vi "Superlight Control.vi"() -> ()   [LabVIEW 2014]
uses:
  statecontrol.ctl
  <vilib>/LabVIEW Interface for Arduino/Type Defs/Board Type.ctl
  <vilib>/LabVIEW Interface for Arduino/Type Defs/Connection Type.ctl
  <vilib>/LabVIEW Interface for Arduino/Type Defs/Pin Mode.ctl
  <vilib>/LabVIEW Interface for Arduino/Type Defs/Arduino Resource.ctl
  <vilib>/LabVIEW Interface for Arduino/LabVIEW Interface for Arduino.lvlib
panel:
  in  "stop 3":bool
  out "high":bool
  out "low":bool
  in  "Power State":bool
  out "Superlight State":T1
  out "cooldown status":bool
  out "Cooldown Time Left":u32 format="%<%M:%S>t"
  out "superlight status":bool
  out "Cooldown Start Time":u32
  in  "stop 2":bool
  out "Superlight On Start Time":u32
  out "Is the button pressed?":bool
  out "Tab Control":enum32{" On", "Off", "CoolDown"}(tab)
  in  "Off":bool
  # "Low"
  # "High"
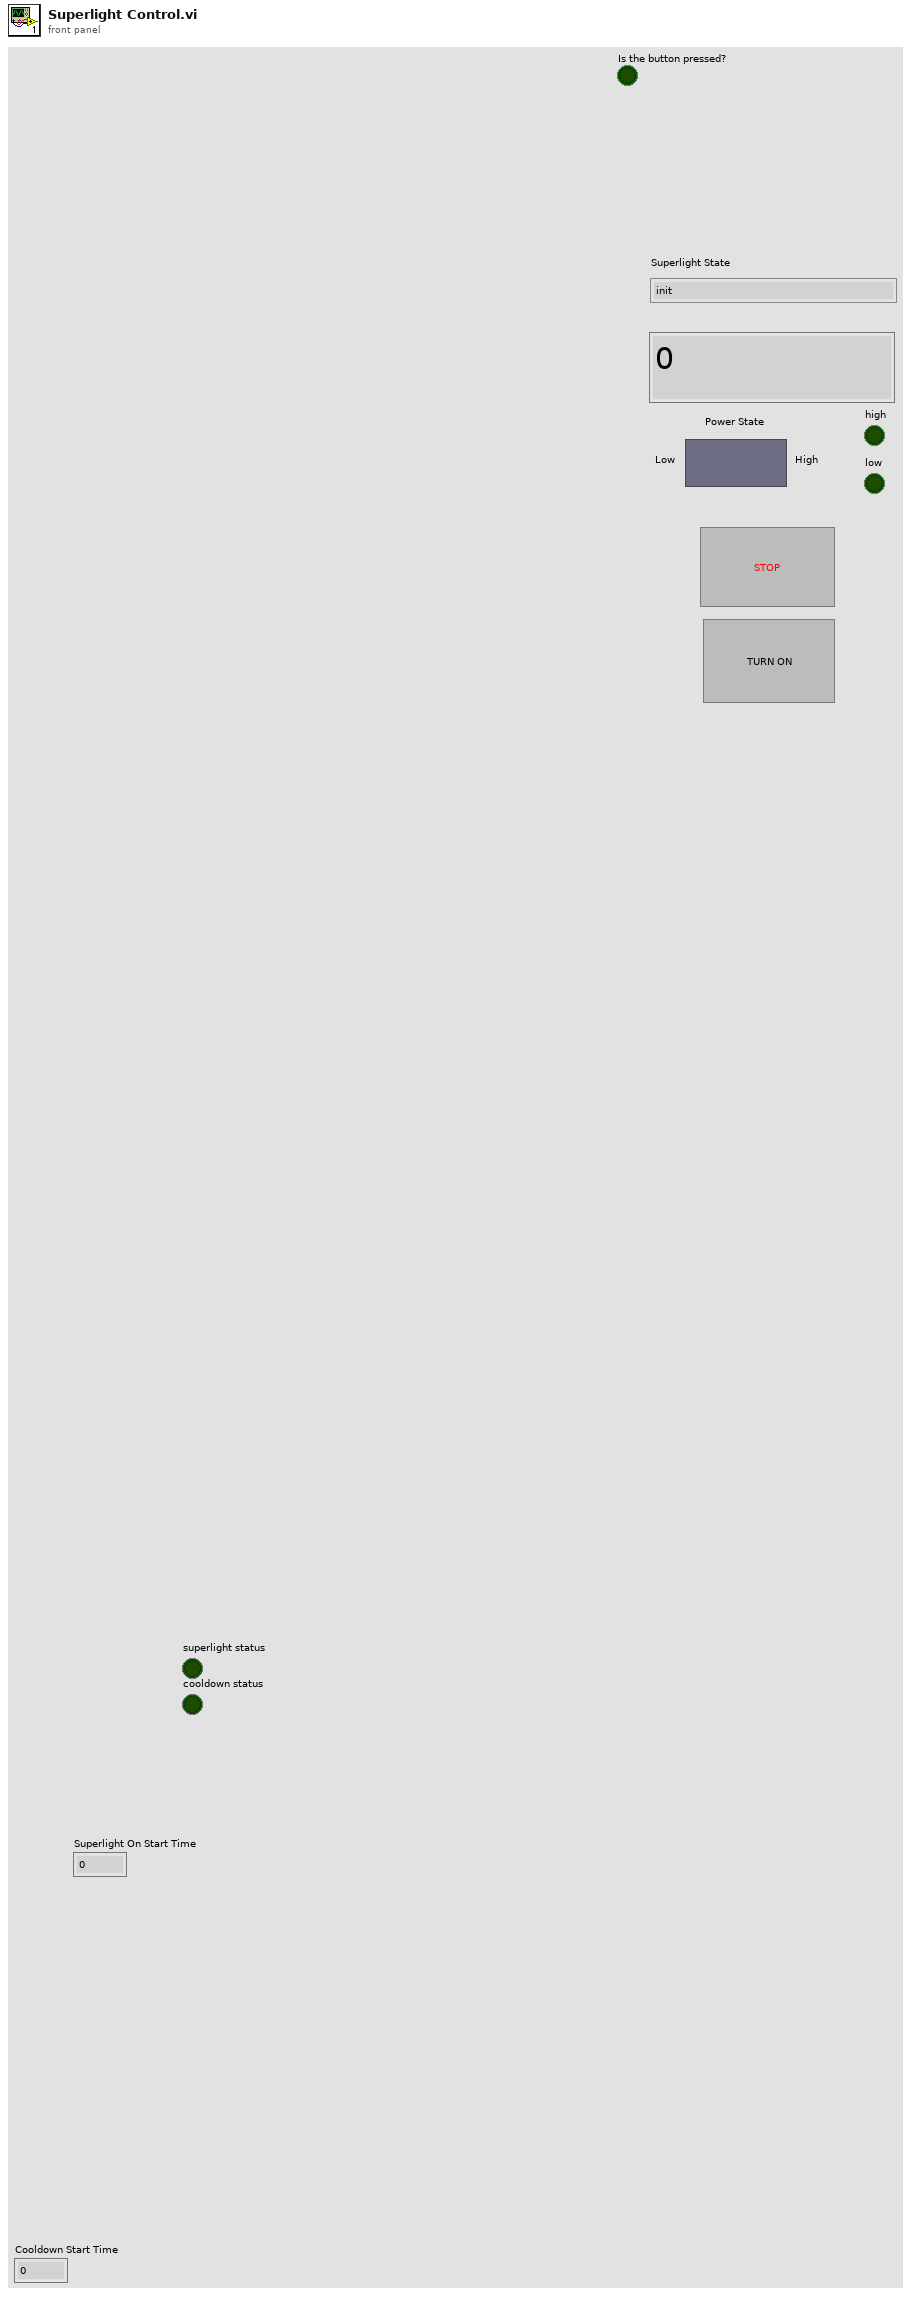
[diagram p1: front panel]
types:
  T1 = typedef "statecontrol.ctl" = enum16{"init", "waiting for trigger", "superlight on", "cooldown", "closing", "shutdown"}
  T2 = typedef "LabVIEW Interface for Arduino.lvlib/Pin Mode.ctl" = enum8{"Input", "Output"}
  T3 = typedef "LabVIEW Interface for Arduino.lvlib/Connection Type.ctl" = enum8{"USB / Serial", "XBEE", "BlueSmirf (Bluetooth)"}
  T4 = typedef "LabVIEW Interface for Arduino.lvlib/Board Type.ctl" = enum16{"Uno", "Dimuelanove w/Atmega 328", "Mega 2560"}
  T5 = typedef "LabVIEW Interface for Arduino.lvlib/Arduino Resource.ctl" = cluster{"VISA resource":refnum<visa-resource-name>, "Board Type":T4, "Connection Type":enum8{"USB / Serial"}, "Bytes Per Packet (15)":u8}
  T6 = enum8{"Enabled", "Disabled", "Disabled and Grayed Out"}
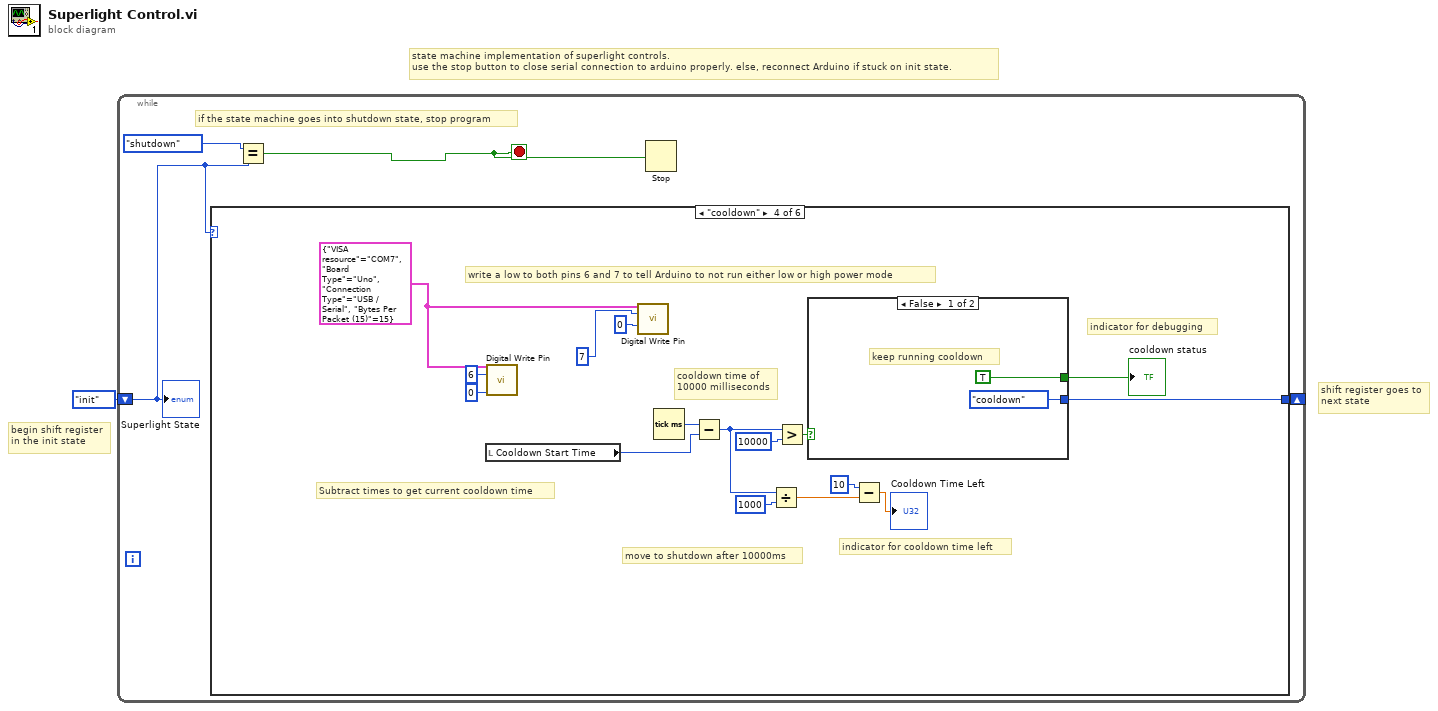
[diagram p0: block diagram]
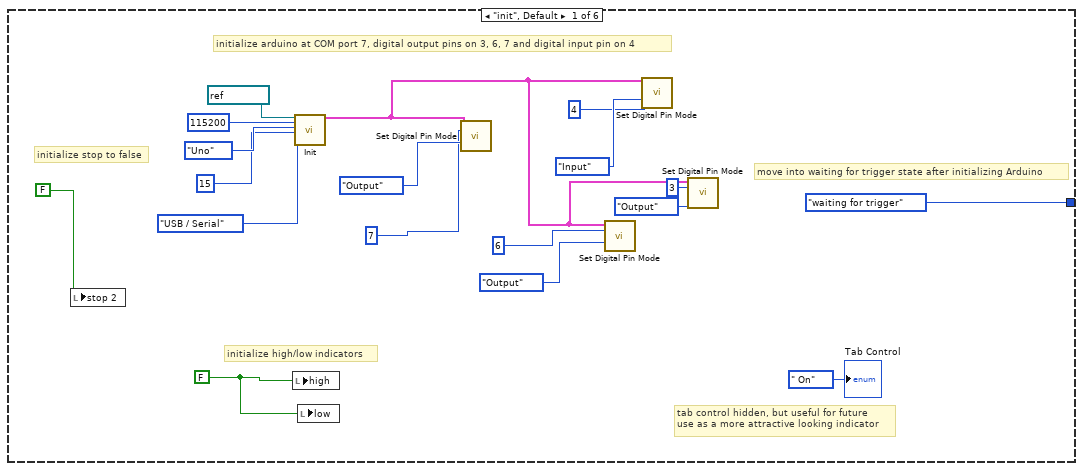
[diagram p2: hidden frame]
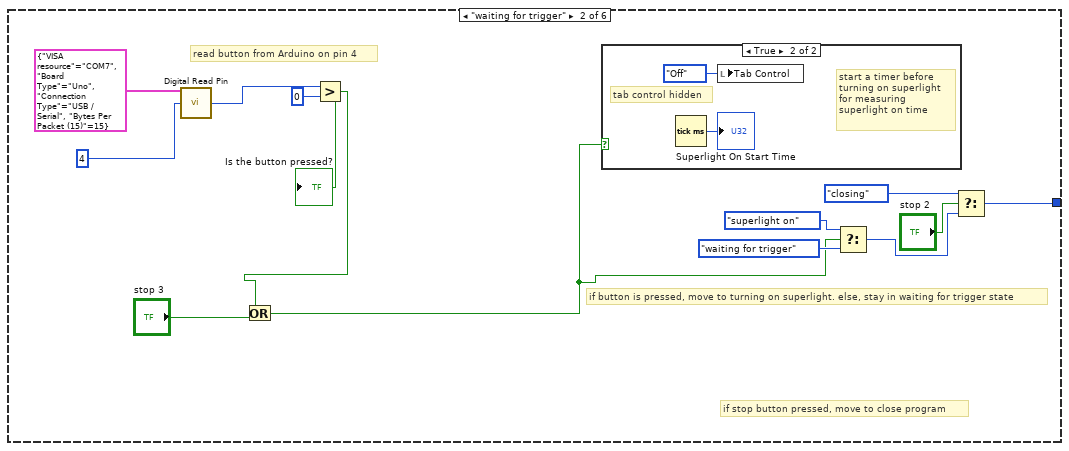
[diagram p3: hidden frame]
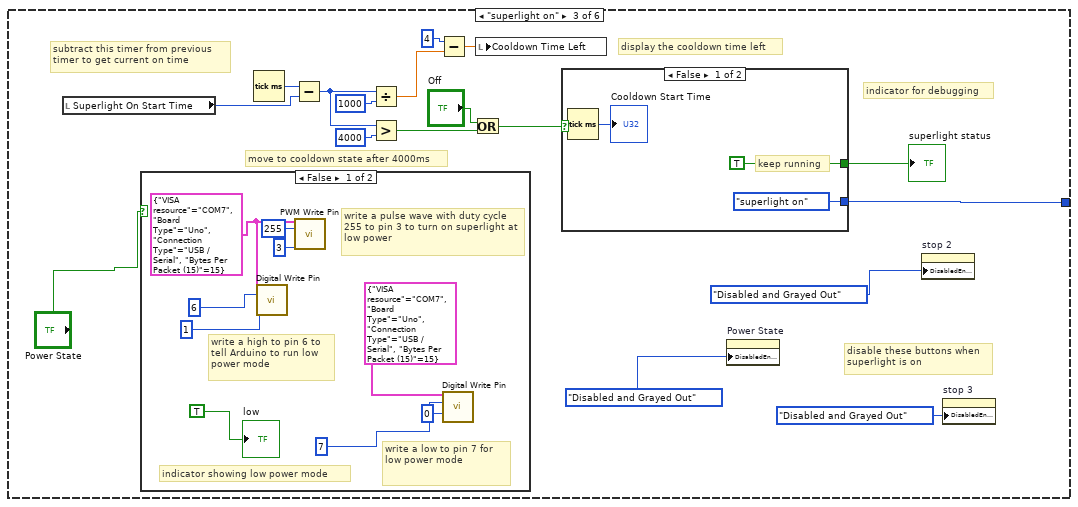
[diagram p5: hidden frame]
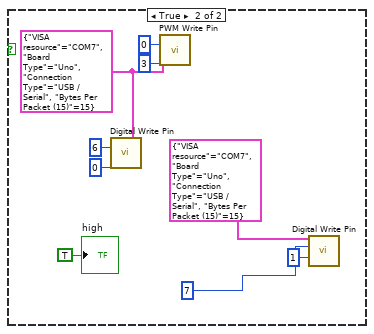
[diagram p6: hidden frame]
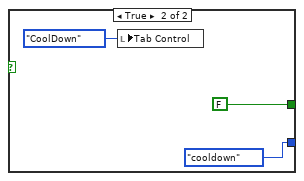
[diagram p7: hidden frame]
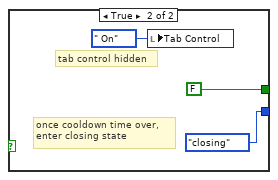
[diagram p8: hidden frame]
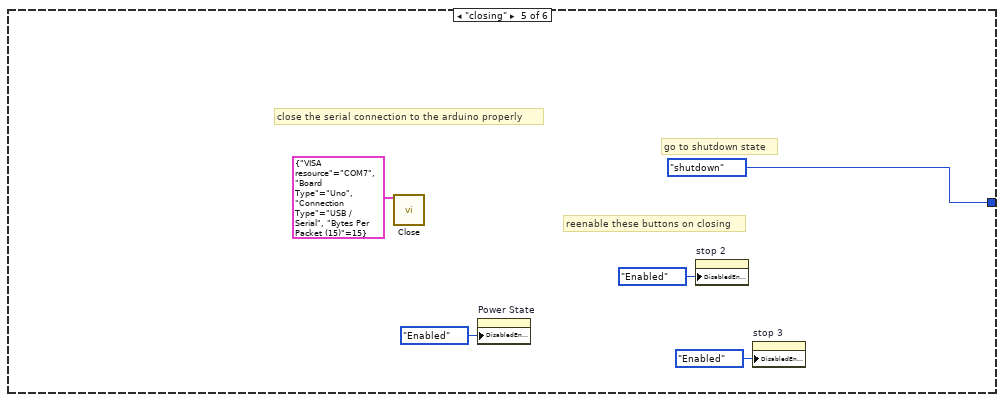
[diagram p9: hidden frame]
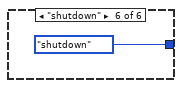
[diagram p10: hidden frame]
diagram:
  # "shift register goes to\nnext state"
  # "begin shift register\nin the init state"
  # "state machine implementation of superlight controls. \nuse the stop button to close serial connection to arduino properly. else, reconnect Arduino if stuck on init state."
  n1 = while {
    shift-right: [w5] -> _
    shift-left: statecontrol."init" ("state") -> [w3]
    stop <- w2 stop-if-true
    # "if the state machine goes into shutdown state, stop program"
    n2 = case shown="\"cooldown\"" w3 {
      tunnel: [statecontrol."waiting for trigger" ("state") w31 w52 w91 statecontrol."shutdown" ("state") statecontrol."shutdown" ("state")] -> w5
      frame "init", Default {
        w6 = FALSE ("high")
        # "tab control hidden, but useful for future \nuse as a more attractive looking indicator"
        # "initialize stop to false"
        # "move into waiting for trigger state after initializing Arduino"
        # "initialize high/low indicators"
        # "initialize arduino at COM port 7, digital output pins on 3, 6, 7 and digital input pin on 4"
        n3 = local write "stop 2"(FALSE ("stop")) -> ()
        n4 = local write "high"(w6) -> ()
        n5 = call <vilib>:"Init.vi"("VISA resource"=refnum<visa-resource-name> "COM7", "Baud Rate (115200)"=u32 115200, "Board Type (Uno)"=Board_Type."Uno", "Bytes Per Packet (15)"=u32 15, "Connection Type (USB/Serial)"=Connection_Type."USB / Serial") -> ("Arduino Resource"=w9:T5)  [unwired: 13 in, 1 out]
        n6 = local write "low"(w6) -> ()
        n7 = call <vilib>:"Set Digital Pin Mode.vi"("Arduino Resource"=w9, "Digital I/O Pin"=u8 7, "Pin Mode (Input)"=Pin_Mode."Output") -> ()  [unwired: 11 in, 2 out]
        n8 = call <vilib>:"Set Digital Pin Mode.vi"("Arduino Resource"=w9, "Digital I/O Pin"=u8 6, "Pin Mode (Input)"=Pin_Mode."Output") -> ()  [unwired: 11 in, 2 out]
        n9 = call <vilib>:"Set Digital Pin Mode.vi"("Arduino Resource"=w9, "Digital I/O Pin"=u8 4, "Pin Mode (Input)"=Pin_Mode."Input") -> ()  [unwired: 11 in, 2 out]
        n10 = call <vilib>:"Set Digital Pin Mode.vi"("Arduino Resource"=w9, "Digital I/O Pin"=u8 3, "Pin Mode (Input)"=Pin_Mode."Output") -> ()  [unwired: 11 in, 2 out]
        "Tab Control" <- enum32{" On", "Off", "CoolDown"}." On" ("Tab Control")
      }
      frame "waiting for trigger" {
        # "if button is pressed, move to turning on superlight. else, stay in waiting for trigger state"
        # "if stop button pressed, move to close program"
        # "read button from Arduino on pin 4"
        n11 = call <vilib>:"Digital Read Pin.vi"("Arduino Resource"=T5 {"VISA resource"="COM7", "Board Type"=enum."Uno", "Connection Type"=enum."USB / Serial", "Bytes Per Packet (15)"=15}, "Digital I/O Pin (0)"=u8 4) -> ("Value"=w28:u8)  [unwired: 11 in, 2 out]
        n12 = Greater?(x=w28, y=u8 0) -> (0:w25:bool)
        "Is the button pressed?" <- w25
        n13 = Or(x=w25, y="stop 3") -> (x .or. y?=w24:bool)
        n14 = case shown="True" w24 {
          frame False {
          }
          frame True {
            # "tab control hidden"
            # "start a timer before\nturning on superlight \nfor measuring \nsuperlight on time"
            n15 = Tick Count (ms)() -> (millisecond timer value=→"Superlight On Start Time":u32)
            n16 = local write "Tab Control"(enum32{" On", "Off", "CoolDown"}."Off" ("Tab Control")) -> ()
          }
        }
        n17 = Select(t=statecontrol."superlight on" ("state"), s=w24, f=statecontrol."waiting for trigger" ("state")) -> (s? t:f=w32:T1)
        n18 = Select(t=statecontrol."closing" ("state"), s="stop 2", f=w32) -> (s? t:f=w31:T1)
      }
      frame "superlight on" {
        # "disable these buttons when\nsuperlight is on"
        # "indicator for debugging"
        # "display the cooldown time left"
        # "subtract this timer from previous \ntimer to get current on time"
        # "move to cooldown state after 4000ms"
        n19 = local read "Superlight On Start Time"() -> (w55:u32)
        n20 = case shown="False" "Power State" {
          frame False {
            w60 = T5 {"VISA resource"="COM7", "Board Type"=enum."Uno", "Connection Type"=enum."USB / Serial", "Bytes Per Packet (15)"=15} ("Arduino Resource")
            # "write a low to pin 7 for low power mode"
            # "indicator showing low power mode"
            # "write a high to pin 6 to \ntell Arduino to run low \npower mode"
            # "write a pulse wave with duty cycle 255 to pin 3 to turn on superlight at low power"
            n21 = call <vilib>:"Digital Write Pin.vi"("Arduino Resource"=w60, "Digital I/O Pin (0)"=u8 6, "Value (0)"=u8 1) -> ()  [unwired: 11 in, 2 out]
            n22 = call <vilib>:"PWM Write Pin.vi"("Arduino Resource"=w60, "Duty Cycle (0 - 255)"=u8 255, "PWM Pin (3)"=u8 3) -> ()  [unwired: 11 in, 2 out]
            n23 = call <vilib>:"Digital Write Pin.vi"("Arduino Resource"=T5 {"VISA resource"="COM7", "Board Type"=enum."Uno", "Connection Type"=enum."USB / Serial", "Bytes Per Packet (15)"=15}, "Digital I/O Pin (0)"=u8 7, "Value (0)"=u8 0) -> ()  [unwired: 11 in, 2 out]
            "low" <- TRUE ("Boolean")
          }
          frame True {
            w71 = T5 {"VISA resource"="COM7", "Board Type"=enum."Uno", "Connection Type"=enum."USB / Serial", "Bytes Per Packet (15)"=15} ("Arduino Resource")
            n24 = call <vilib>:"Digital Write Pin.vi"("Arduino Resource"=w71, "Digital I/O Pin (0)"=u8 6, "Value (0)"=u8 0) -> ()  [unwired: 11 in, 2 out]
            n25 = call <vilib>:"PWM Write Pin.vi"("Arduino Resource"=w71, "Duty Cycle (0 - 255)"=u8 0, "PWM Pin (3)"=u8 3) -> ()  [unwired: 11 in, 2 out]
            n26 = call <vilib>:"Digital Write Pin.vi"("Arduino Resource"=T5 {"VISA resource"="COM7", "Board Type"=enum."Uno", "Connection Type"=enum."USB / Serial", "Bytes Per Packet (15)"=15}, "Digital I/O Pin (0)"=u8 7, "Value (0)"=u8 1) -> ()  [unwired: 11 in, 2 out]
            "high" <- TRUE ("Boolean 2")
          }
        }
        n27 = Tick Count (ms)() -> (millisecond timer value=w54:u32)
        n28 = Subtract(x=w54, y=w55) -> (x-y=w43:u32)
        n29 = Divide(x=w43, y=u32 1000) -> (x/y=w49:dbl)
        n30 = Greater?(x=w43, y=u32 4000) -> (0:w46:bool)
        n31 = Subtract(x=u32 4, y=w49) -> (x-y=w44:dbl)
        n32 = Or(x="Off", y=w46) -> (x .or. y?=w45:bool)
        n33 = local write "Cooldown Time Left"(w44) -> ()
        n34 = case shown="False" w45 {
          tunnel: [TRUE FALSE] -> w53
          tunnel: [statecontrol."superlight on" ("state") statecontrol."cooldown" ("state")] -> w52
          frame False {
            # "keep running"
            n35 = Tick Count (ms)() -> (millisecond timer value=→"Cooldown Start Time":u32)
          }
          frame True {
            n36 = local write "Tab Control"(enum32{" On", "Off", "CoolDown"}."CoolDown" ("Tab Control")) -> ()
          }
        }
        "superlight status" <- w53
        n37 = property on="Power State" class="Bool (strict)"("DisabledEnum"=T6."Disabled and Grayed Out" ("Disabled")) -> ()  [unwired: 2 in, 2 out]
        n38 = property on="stop 2" class="Bool (strict)"("DisabledEnum"=T6."Disabled and Grayed Out" ("Disabled")) -> ()  [unwired: 2 in, 2 out]
        n39 = property on="stop 3" class="Bool"("DisabledEnum"=T6."Disabled and Grayed Out" ("Disabled")) -> ()  [unwired: 2 in, 2 out]
      }
      frame "cooldown" {
        w80 = T5 {"VISA resource"="COM7", "Board Type"=enum."Uno", "Connection Type"=enum."USB / Serial", "Bytes Per Packet (15)"=15} ("Arduino Resource")
        # "indicator for cooldown time left"
        # "indicator for debugging"
        # "Subtract times to get current cooldown time"
        # "cooldown time of \n10000 milliseconds"
        # "write a low to both pins 6 and 7 to tell Arduino to not run either low or high power mode"
        # "move to shutdown after 10000ms"
        n40 = local read "Cooldown Start Time"() -> (w95:u32)
        n41 = call <vilib>:"Digital Write Pin.vi"("Arduino Resource"=w80, "Digital I/O Pin (0)"=u8 6, "Value (0)"=u8 0) -> ()  [unwired: 11 in, 2 out]
        n42 = call <vilib>:"Digital Write Pin.vi"("Arduino Resource"=w80, "Digital I/O Pin (0)"=u8 7, "Value (0)"=u8 0) -> ()  [unwired: 11 in, 2 out]
        n43 = Tick Count (ms)() -> (millisecond timer value=w94:u32)
        n44 = Subtract(x=w94, y=w95) -> (x-y=w87:u32)
        n45 = Divide(x=w87, y=u32 1000) -> (x/y=w88:dbl)
        n46 = Greater?(x=w87, y=u32 10000) -> (0:w93:bool)
        n47 = case shown="False" w93 {
          tunnel: [TRUE FALSE] -> w92
          tunnel: [statecontrol."cooldown" ("state") statecontrol."closing" ("state")] -> w91
          frame False {
            # "keep running cooldown"
          }
          frame True {
            # "tab control hidden"
            # "once cooldown time over,\nenter closing state"
            n48 = local write "Tab Control"(enum32{" On", "Off", "CoolDown"}." On" ("Tab Control")) -> ()
          }
        }
        "cooldown status" <- w92
        n49 = Subtract(x=u32 10, y=w88) -> (x-y=→"Cooldown Time Left":dbl)
      }
      frame "closing" {
        # "reenable these buttons on closing"
        # "go to shutdown state"
        # "close the serial connection to the arduino properly"
        n50 = call <vilib>:"Close.vi"("Arduino Resource"=T5 {"VISA resource"="COM7", "Board Type"=enum."Uno", "Connection Type"=enum."USB / Serial", "Bytes Per Packet (15)"=15}) -> ()  [unwired: 14 in, 1 out]
        n51 = property on="Power State" class="Bool (strict)"("DisabledEnum"=T6."Enabled" ("Disabled")) -> ()  [unwired: 2 in, 2 out]
        n52 = property on="stop 2" class="Bool (strict)"("DisabledEnum"=T6."Enabled" ("Disabled")) -> ()  [unwired: 2 in, 2 out]
        n53 = property on="stop 3" class="Bool"("DisabledEnum"=T6."Enabled" ("Disabled")) -> ()  [unwired: 2 in, 2 out]
      }
      frame "shutdown" {
      }
    }
    n54 = Equal?(x=statecontrol."shutdown" ("state"), y=w3) -> (x = y?=w2:bool)
    n55 = Stop(stop? (T)=w2) -> ()
    "Superlight State" <- w3
  }
